vi "Unit Test VI.vi"() -> ()   [LabVIEW 2017]
uses:
  PPLs/Power Supply/Parent/Power_Supply.lvlibp/Custom Control/Supply Settings.ctl
  N5745A.lvclass
  PPLs/Power Supply/Parent/Power_Supply.lvlibp/Custom Control/Protection.ctl
  PPLs/Power Supply/Parent/Power_Supply.lvlibp/Power Supply.lvclass
  C:/Projects/LabVIEW/PPLs/Power Supply/Parent/Power_Supply.lvlibp/Power Supply.lvclass
  PPLs/Power Supply/Parent/Power_Supply.lvlibp
panel:
  in  "Limit":dbl format="%.2f"
  in  "Protection (None)":T1=enum."Over Current"
  out "Output":bool
  out "Current":dbl format="%.6f"
  out "Voltage":dbl format="%.6f"
  in  "Lock?":bool
  out "error out":errorcluster
  in  "N5745A in":refnum<class "N5745A.lvclass">
  in  "Resource":refnum<visa-resource-name>="TCPIP0::169.254.57.0::inst0::INSTR"
  in  "Settings":T2
  in  "error in (no error)":errorcluster
  # "1. Provide Resource ID - Defaults to LAN IP Address for N5745A.\n2. Provide Voltage, Current and Output settings.\n3. Set Protection. Set Limit if seetting OVP & UVL. Setting OCP ignores the Limit field.\n4. Choose to lock front panel buttons and knobs. Run VI"
  # "1."
  # "2."
  # "3."
  # "4."
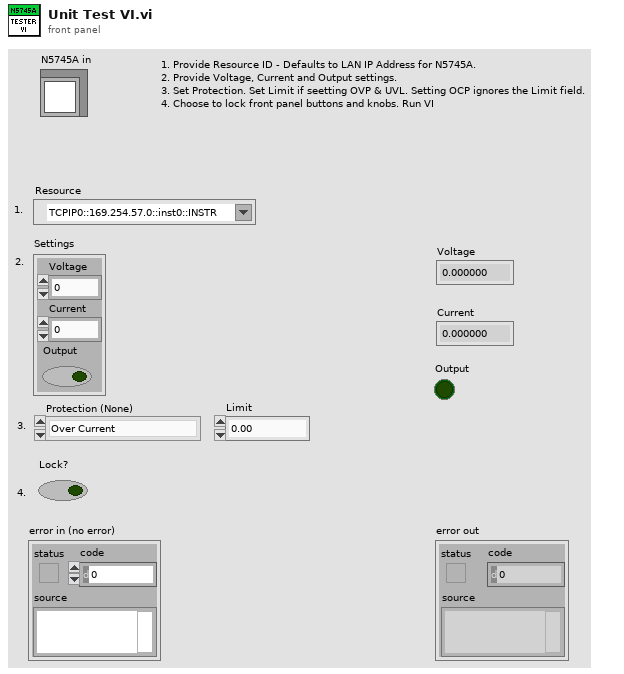
[diagram p1: front panel]
types:
  T1 = typedef "Power_Supply.lvlibp/Protection.ctl" = enum16{"None", "Over Volt", "Under Volt", "Over Current"}
  T2 = typedef "Power_Supply.lvlibp/Supply Settings.ctl" = cluster{"Voltage":dbl, "Current":dbl, "Output":bool}
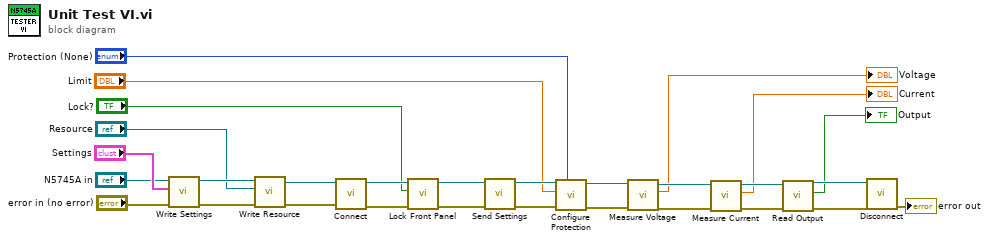
[diagram p0: block diagram]
diagram:
  n1 = call "Write Settings.vi"("error in (no error)"="error in (no error)", "Settings"="Settings", "Power Supply in"="N5745A in") -> ("error out"=w26:errorcluster, "Power Supply out"=w27:refnum<class "N5745A.lvclass">)  [unwired: 7 in]
  n2 = call "Write Resource.vi"("error in"=w26, "Resource"="Resource", "Power Supply in"=w27) -> ("error out"=w21:errorcluster, "Power Supply out"=w22:refnum<class "N5745A.lvclass">)  [unwired: 7 in]
  n3 = call-dynamic "Connect.vi"("error in (no error)"=w21, "N5745A in"=w22) -> ("error out"=w19:errorcluster, "N5745A out"=w20:refnum<class "N5745A.lvclass">)  [unwired: 8 in]
  n4 = call-dynamic "Lock Front Panel.vi"("error in (no error)"=w19, "Lock?"="Lock?", "N5745A in"=w20) -> ("error out"=w17:errorcluster, "N5745A out"=w18:refnum<class "N5745A.lvclass">)  [unwired: 7 in]
  n5 = call-dynamic "Send Settings.vi"("error in (no error)"=w17, "N5745A in"=w18) -> ("error out"=w13:errorcluster, "N5745A out"=w15:refnum<class "N5745A.lvclass">)  [unwired: 8 in]
  n6 = call-dynamic "Configure Protection.vi"("Protection (None)"="Protection (None)", "error in (no error)"=w13, "Limit"="Limit", "N5745A in"=w15) -> ("error out"=w5:errorcluster, "N5745A out"=w6:refnum<class "N5745A.lvclass">)  [unwired: 6 in]
  n7 = call-dynamic "Measure Voltage.vi"("error in (no error)"=w5, "N5745A in"=w6) -> ("error out"=w9:errorcluster, "Voltage"=→"Voltage":dbl, "N5745A out"=w12:refnum<class "N5745A.lvclass">)  [unwired: 7 in]
  n8 = call-dynamic "Measure Current.vi"("error in (no error)"=w9, "N5745A in"=w12) -> ("error out"=w10:errorcluster, "Current"=→"Current":dbl, "N5745A out"=w11:refnum<class "N5745A.lvclass">)  [unwired: 7 in]
  n9 = call-dynamic "Read Output.vi"("error in"=w10, "N5745A in"=w11) -> ("error out"=w8:errorcluster, "Output"=→"Output":bool, "N5745A out"=w7:refnum<class "N5745A.lvclass">)  [unwired: 7 in]
  n10 = call-dynamic "Disconnect.vi"("error in (no error)"=w8, "N5745A in"=w7) -> ("error out"=→"error out":errorcluster)  [unwired: 8 in, 1 out]
